vi "json_example.vi"(8 "error in (no error)":errorcluster) -> (0 "error out":errorcluster, 2 "flattened variant":variant, 10 "nested variant":variant)   [LabVIEW 2011]
doc: "An example of how to use the parse, flatten, and scriptCluster VI's."
panel:
  in  "Script clusters?":bool
  in  "json string":string="{\"bob\":\"aabner\",\n\"bool\":false,\n\"number\":1.2,\n\"arrg\":[1,2,3]}"
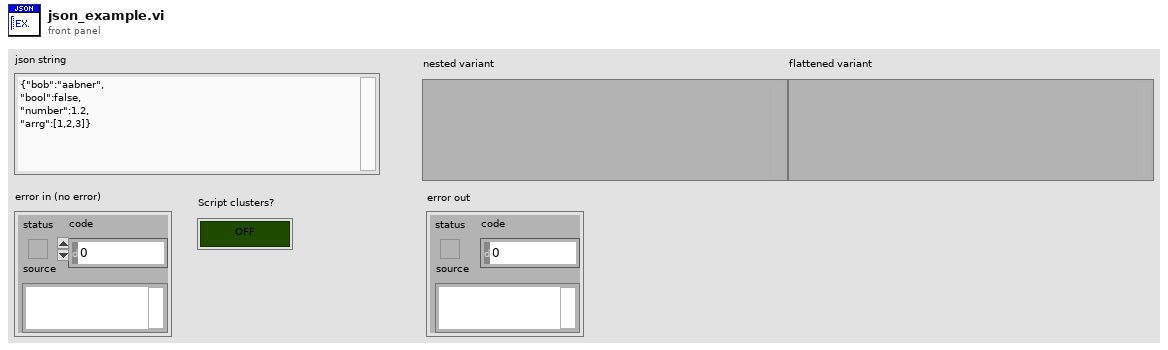
[diagram p1: front panel]
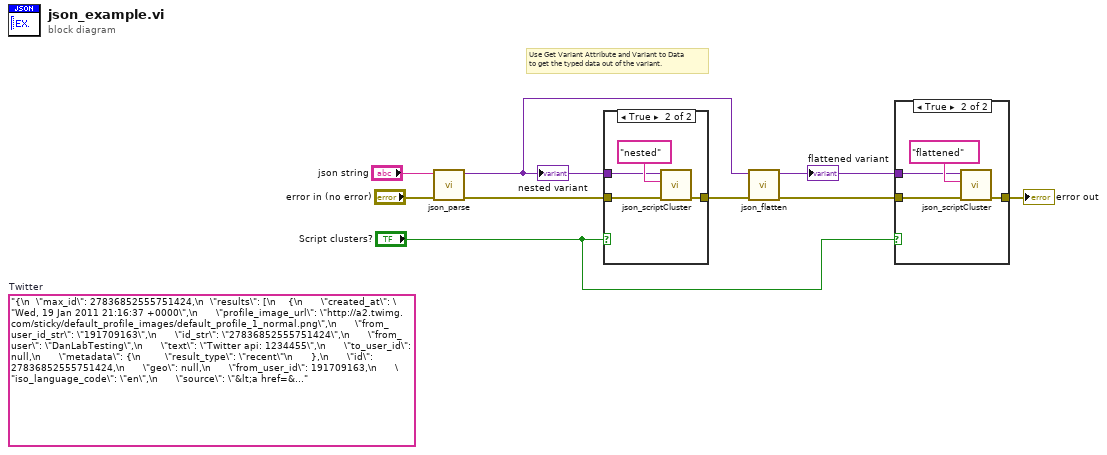
[diagram p0: block diagram]
diagram:
  (unwired) "{\n  \"max_id\": 27836852555751424,\n  \"results\": [\n    {\n      \"created_at\": \"Wed, 19 Jan 2011 21:16:37 +0000\",\n      \"profile_image_url\": \"http://a2.twimg.com/sticky/default_profile_images/default_profile_1_normal.png\",\n      \"from_user_id_str\": \"191709163\",\n      \"id_str\": \"27836852555751424\",\n      \"from_user\": \"DanLabTesting\",\n      \"text\": \"Twitter api: 1234455\",\n      \"to_user_id\": null,\n      \"metadata\": {\n        \"result_type\": \"recent\"\n      },\n      \"id\": 27836852555751424,\n      \"geo\": null,\n      \"from_user_id\": 191709163,\n      \"iso_language_code\": \"en\",\n      \"source\": \"&lt;a href=&quot;http://www.danlabgames.com/index.php?computer=ipad&quot; rel=&quot;nofollow&quot;&gt;Wacka Monsta&lt;/a&gt;\",\n      \"to_user_id_str\": null\n    },\n    {\n      \"created_at\": \"Wed, 19 Jan 2011 21:12:02 +0000\",\n      \"profile_image_url\": \"http://a0.twimg.com/profile_images/1142619698/DSC_0195_normal.jpg\",\n      \"from_user_id_str\": \"165544885\",\n      \"id_str\": \"27835698383945728\",\n      \"from_user\": \"Deberamatkin\",\n      \"text\": \"Fetching the number of followers without using any Twitter API http://pr9.in/4q\",\n      \"to_user_id\": null,\n      \"metadata\": {\n        \"result_type\": \"recent\"\n      },\n      \"id\": 27835698383945728,\n      \"geo\": null,\n      \"from_user_id\": 165544885,\n      \"iso_language_code\": \"en\",\n      \"source\": \"&lt;a href=&quot;http://www.exaspring.com&quot; rel=&quot;nofollow&quot;&gt;ExaSpring Information Services&lt;/a&gt;\",\n      \"to_user_id_str\": null\n    },\n    {\n      \"created_at\": \"Wed, 19 Jan 2011 20:57:35 +0000\",\n      \"profile_image_url\": \"http://a3.twimg.com/profile_images/1093562803/__F1000040mini_normal.jpg\",\n      \"from_user_id_str\": \"95281337\",\n      \"id_str\": \"27832064640290817\",\n      \"from_user\": \"Lito_tweet\",\n      \"text\": \"More info can be found here http://support.twitter.com/articles/15364-about-twitter-limits-update-api-dm-and-following\",\n      \"to_user_id\": null,\n      \"metadata\": {\n        \"result_type\": \"recent\"\n      },\n      \"id\": 27832064640290817,\n      \"geo\": null,\n      \"from_user_id\": 95281337,\n      \"iso_language_code\": \"en\",\n      \"source\": \"&lt;a href=&quot;http://yubitter.com/&quot; rel=&quot;nofollow&quot;&gt;yubitter&lt;/a&gt;\",\n      \"to_user_id_str\": null\n    },\n    {\n      \"created_at\": \"Wed, 19 Jan 2011 20:53:18 +0000\",\n      \"profile_image_url\": \"http://a1.twimg.com/profile_images/1196625301/Twitter_normal.JPG\",\n      \"from_user_id_str\": \"77719707\",\n      \"id_str\": \"27830982988005377\",\n      \"from_user\": \"g_a_x\",\n      \"text\": \"RT @ramirezviki: RT @g_a_x: &quot;Twitter Status: Twitter API rate excedeed&quot; WTF??? // Que dejes de twittearrrr!!!!!!!!!!!  // JJAJAJAJAJJAAA\",\n      \"to_user_id\": null,\n      \"metadata\": {\n        \"result_type\": \"recent\"\n      },\n      \"id\": 27830982988005377,\n      \"geo\": null,\n      \"from_user_id\": 77719707,\n      \"iso_language_code\": \"en\",\n      \"source\": \"&lt;a href=&quot;http://www.tweetdeck.com&quot; rel=&quot;nofollow&quot;&gt;TweetDeck&lt;/a&gt;\",\n      \"to_user_id_str\": null\n    },\n    {\n      \"created_at\": \"Wed, 19 Jan 2011 20:51:06 +0000\",\n      \"profile_image_url\": \"http://a2.twimg.com/profile_images/673715309/danlablogo_normal.png\",\n      \"from_user_id_str\": \"20913275\",\n      \"id_str\": \"27830431516729344\",\n      \"from_user\": \"DanLabGames\",\n      \"text\": \"Working on Facebook and Twitter API on iPhone.. Silly Piece of code. But it Work\",\n      \"to_user_id\": null,\n      \"metadata\": {\n        \"result_type\": \"recent\"\n      },\n      \"id\": 27830431516729344,\n      \"geo\": null,\n      \"from_user_id\": 20913275,\n      \"iso_language_code\": \"en\",\n      \"source\": \"&lt;a href=&quot;http://www.danlabgames.com/index.php?computer=ipad&quot; rel=&quot;nofollow&quot;&gt;Wacka Monsta&lt;/a&gt;\",\n      \"to_user_id_str\": null\n    },\n    {\n      \"created_at\": \"Wed, 19 Jan 2011 20:44:42 +0000\",\n      \"profile_image_url\": \"http://a1.twimg.com/profile_images/1220195008/BeautyIsHerName_normal.JPG\",\n      \"from_user_id_str\": \"180040602\",\n      \"id_str\": \"27828818869747713\",\n      \"from_user\": \"MozBWanKinobi\",\n      \"text\": \"@Patroose It's slow as shit, that damn Twitter API thing pops up every 5 minutes, and won't post tweets half the time, they need to fix it\",\n      \"to_user_id\": 16219315,\n      \"metadata\": {\n        \"result_type\": \"recent\"\n      },\n      \"id\": 27828818869747713,\n      \"geo\": null,\n      \"to_user\": \"Patroose\",\n      \"from_user_id\": 180040602,\n      \"iso_language_code\": \"en\",\n      \"source\": \"&lt;a href=&quot;http://twitter.com/&quot;&gt;web&lt;/a&gt;\",\n      \"to_user_id_str\": \"16219315\"\n    },\n    {\n      \"created_at\": \"Wed, 19 Jan 2011 20:42:13 +0000\",\n      \"profile_image_url\": \"http://a3.twimg.com/profile_images/1167064690/b460f7b0-d6ac-4d8a-b025-998cadb31acc_normal.png\",\n      \"from_user_id_str\": \"11861298\",\n      \"id_str\": \"27828194379833345\",\n      \"from_user\": \"twittwootwiggy\",\n      \"text\": \"@USoBritain @elejamie Cheers, if i'm on the list i will prove i'm worth it. http://api.twitter.com/EDLinfidel/wankers#\",\n      \"to_user_id\": 105839068,\n      \"metadata\": {\n        \"result_type\": \"recent\"\n      },\n      \"id\": 27828194379833345,\n      \"geo\": null,\n      \"to_user\": \"USoBritain\",\n      \"from_user_id\": 11861298,\n      \"iso_language_code\": \"en\",\n      \"source\": \"&lt;a href=&quot;http://twitter.com/&quot;&gt;web&lt;/a&gt;\",\n      \"to_user_id_str\": \"105839068\"\n    },\n    {\n      \"created_at\": \"Wed, 19 Jan 2011 20:35:29 +0000\",\n      \"profile_image_url\": \"http://a2.twimg.com/profile_images/1197946386/Seb_lasLe_as_normal.jpg\",\n      \"from_user_id_str\": \"155070729\",\n      \"id_str\": \"27826502271762432\",\n      \"from_user\": \"iSebx\",\n      \"text\": \"RT @g_a_x &quot;Twitter Status: Twitter API rate excedeed&quot; WTF??? // estaba por postear lo mismo no me dejaba subir una foto\",\n      \"to_user_id\": null,\n      \"metadata\": {\n        \"result_type\": \"recent\"\n      },\n      \"id\": 27826502271762432,\n      \"geo\": null,\n      \"from_user_id\": 155070729,\n      \"iso_language_code\": \"en\",\n      \"source\": \"&lt;a href=&quot;http://www.tweetdeck.com&quot; rel=&quot;nofollow&quot;&gt;TweetDeck&lt;/a&gt;\",\n      \"to_user_id_str\": null\n    },\n    {\n      \"created_at\": \"Wed, 19 Jan 2011 20:24:26 +0000\",\n      \"profile_image_url\": \"http://a2.twimg.com/profile_images/859603564/johannes_normal.jpg\",\n      \"from_user_id_str\": \"104685382\",\n      \"id_str\": \"27823718839361536\",\n      \"from_user\": \"seo_depp\",\n      \"text\": \"rt @davide_rosi2011#analytics New ActionScript 3 Library For The API: We love simplifying access to Google Analy... http://bit.ly/i8k0IA\",\n      \"to_user_id\": null,\n      \"metadata\": {\n        \"result_type\": \"recent\"\n      },\n      \"id\": 27823718839361536,\n      \"geo\": null,\n      \"from_user_id\": 104685382,\n      \"iso_language_code\": \"en\",\n      \"source\": \"&lt;a href=&quot;http://twitterfeed.com&quot; rel=&quot;nofollow&quot;&gt;twitterfeed&lt;/a&gt;\",\n      \"to_user_id_str\": null\n    },\n    {\n      \"created_at\": \"Wed, 19 Jan 2011 20:21:46 +0000\",\n      \"profile_image_url\": \"http://a1.twimg.com/profile_images/1196625301/Twitter_normal.JPG\",\n      \"from_user_id_str\": \"77719707\",\n      \"id_str\": \"27823049667510272\",\n      \"from_user\": \"g_a_x\",\n      \"text\": \"&quot;Twitter Status: Twitter API rate excedeed&quot; WTF???\",\n      \"to_user_id\": null,\n      \"metadata\": {\n        \"result_type\": \"recent\"\n      },\n      \"id\": 27823049667510272,\n      \"geo\": null,\n      \"from_user_id\": 77719707,\n      \"iso_language_code\": \"en\",\n      \"source\": \"&lt;a href=&quot;http://www.tweetdeck.com&quot; rel=&quot;nofollow&quot;&gt;TweetDeck&lt;/a&gt;\",\n      \"to_user_id_str\": null\n    },\n    {\n      \"created_at\": \"Wed, 19 Jan 2011 20:05:22 +0000\",\n      \"profile_image_url\": \"http://a1.twimg.com/profile_images/1102380575/61918c9a-8d5c-4390-b41f-b234398cd5d4_normal.png\",\n      \"from_user_id_str\": \"7654007\",\n      \"id_str\": \"27818920278757376\",\n      \"from_user\": \"ConMend\",\n      \"text\": \"#TwitterHelp #Help #CallingofTheGeeks Please help me get rid of the Twitter API dialogue box that pops up every bleeding minute!\",\n      \"to_user_id\": null,\n      \"metadata\": {\n        \"result_type\": \"recent\"\n      },\n      \"id\": 27818920278757376,\n      \"geo\": null,\n      \"from_user_id\": 7654007,\n      \"iso_language_code\": \"en\",\n      \"source\": \"&lt;a href=&quot;http://twitter.com/&quot;&gt;web&lt;/a&gt;\",\n      \"to_user_id_str\": null\n    },\n    {\n      \"created_at\": \"Wed, 19 Jan 2011 19:55:36 +0000\",\n      \"profile_image_url\": \"http://a3.twimg.com/profile_images/1167064690/b460f7b0-d6ac-4d8a-b025-998cadb31acc_normal.png\",\n      \"from_user_id_str\": \"11861298\",\n      \"id_str\": \"27816463830089728\",\n      \"from_user\": \"twittwootwiggy\",\n      \"text\": \"Its easy to get on http://api.twitter.com/#!/EDLinfidel/wankers @Andrea_UrbanFox just ask @EDLinfidel a Hypothetical question referring #EDL\",\n      \"to_user_id\": null,\n      \"metadata\": {\n        \"result_type\": \"recent\"\n      },\n      \"id\": 27816463830089728,\n      \"geo\": null,\n      \"from_user_id\": 11861298,\n      \"iso_language_code\": \"en\",\n      \"source\": \"&lt;a href=&quot;http://twitter.com/&quot;&gt;web&lt;/a&gt;\",\n      \"to_user_id_str\": null\n    },\n    {\n      \"created_at\": \"Wed, 19 Jan 2011 19:55:10 +0000\",\n      \"profile_image_url\": \"http://a0.twimg.com/profile_images/585494683/13038_613894593395_24403188_35452430_7524658_n_normal.jpg\",\n      \"from_user_id_str\": \"1493373\",\n      \"id_str\": \"27816354073550848\",\n      \"from_user\": \"mirandafte\",\n      \"text\": \"@mirandafte testing some twitter API - ness\",\n      \"to_user_id\": 1493373,\n      \"metadata\": {\n        \"result_type\": \"recent\"\n      },\n      \"id\": 27816354073550848,\n      \"geo\": null,\n      \"to_user\": \"mirandafte\",\n      \"from_user_id\": 1493373,\n      \"iso_language_code\": \"en\",\n      \"source\": \"&lt;a href=&quot;http://twitter.com/&quot;&gt;web&lt;/a&gt;\",\n      \"to_user_id_str\": \"1493373\"\n    },\n    {\n      \"created_at\": \"Wed, 19 Jan 2011 19:55:07 +0000\",\n      \"profile_image_url\": \"http://a0.twimg.com/profile_images/1213136572/110105-195452_normal.jpg\",\n      \"from_user_id_str\": \"134087646\",\n      \"id_str\": \"27816342371434496\",\n      \"from_user\": \"rachel8973\",\n      \"text\": \"Actually @TweetDeck it's not your fault it's the useless @twitter API. But you still smell\",\n      \"to_user_id\": null,\n      \"metadata\": {\n        \"result_type\": \"recent\"\n      },\n      \"id\": 27816342371434496,\n      \"geo\": null,\n      \"from_user_id\": 134087646,\n      \"iso_language_code\": \"en\",\n      \"source\": \"&lt;a href=&quot;http://seesmic.com/app&quot; rel=&quot;nofollow&quot;&gt;Seesmic Web&lt;/a&gt;\",\n      \"to_user_id_str\": null\n    },\n    {\n      \"created_at\": \"Wed, 19 Jan 2011 19:52:39 +0000\",\n      \"profile_image_url\": \"http://a3.twimg.com/profile_images/1172946788/eagle-flag-4_normal.jpg\",\n      \"from_user_id_str\": \"174036699\",\n      \"id_str\": \"27815721295679488\",\n      \"from_user\": \"benny_hans\",\n      \"text\": \"One Reason For Those Twitter API Limits: Search Volume is Soaring http://bit.ly/aksMW2 #twitter #twittertips\",\n      \"to_user_id\": null,\n      \"metadata\": {\n        \"result_type\": \"recent\"\n      },\n      \"id\": 27815721295679488,\n      \"geo\": null,\n      \"from_user_id\": 174036699,\n      \"iso_language_code\": \"en\",\n      \"source\": \"&lt;a href=&quot;http://twitter.com/&quot;&gt;web&lt;/a&gt;\",\n      \"to_user_id_str\": null\n    }\n  ],\n  \"since_id\": 0,\n  \"refresh_url\": \"?since_id=27836852555751424&q=Twitter+API\",\n  \"next_page\": \"?page=2&max_id=27836852555751424&q=Twitter+API\",\n  \"page\": 1,\n  \"results_per_page\": 15,\n  \"completed_in\": 0.075744,\n  \"since_id_str\": \"0\",\n  \"query\": \"Twitter+API\",\n  \"max_id_str\": \"27836852555751424\"\n}"  # Twitter
  # "Use Get Variant Attribute and Variant to Data\nto get the typed data out of the variant."
  n1 = call "json_parse.vi"("error in (no error)"="error in (no error)", "source"="json string") -> ("error out"=w6:errorcluster, "value"=w5:variant)  [unwired: 8 in]
  "nested variant" <- w5
  n2 = case shown="True" "Script clusters?" {
    tunnel: [w10 w13] -> w7
    tunnel: w6 -> [w10 w12]
    tunnel: w5 -> [_ w11]
    frame False {
    }
    frame True {
      n3 = call "json_scriptCluster.vi"("error in (no error)"=w12, "cluster label"="nested", "json variant"=w11) -> ("error out"=w13:errorcluster)  [unwired: 8 in]
    }
  }
  n4 = call "json_flatten.vi"("error in (no error)"=w7, "json variant"=w5) -> ("error out"=w4:errorcluster, "flattened variant"=w3:variant)  [unwired: 8 in]
  "flattened variant" <- w3
  n5 = case shown="True" "Script clusters?" {
    tunnel: w4 -> [w15 w18]
    tunnel: w3 -> [_ w17]
    tunnel: [w15 w16] -> w2
    frame False {
    }
    frame True {
      n6 = call "json_scriptCluster.vi"("error in (no error)"=w18, "cluster label"="flattened", "json variant"=w17) -> ("error out"=w16:errorcluster)  [unwired: 8 in]
    }
  }
  "error out" <- w2
